vi "PCB name at location.vi"(0 "PCB Outlines in":T1(array[cluster]), 1 "XY Graph":refnum<vi>, 7 "XY":cluster{"X":dbl, "Y":dbl}, 11 "error in":errorcluster) -> (4 "PCB Outlines out":T1(array[cluster]), 6 "PCB Name":string, 8 "Outline mean":cluster{"X":dbl, "Y":dbl}, 10 "Within outline":bool, 14 "x y position":cluster{"X":dbl, "Y":dbl}, 15 "error out":errorcluster)   [LabVIEW 2013, in "Manipulate IPF.lvlib"]
uses:
  <vilib>/Analysis/baseanly.llb/Mean (DBL).vi
  <vilib>/Analysis/geometry.llb/Point in Polygon (Scalar).vi
  Manipulate IPF.lvlib
  <vilib>/Analysis/NI_AAL_Geometry.lvlib
  <vilib>/Analysis/NI_AALBase.lvlib
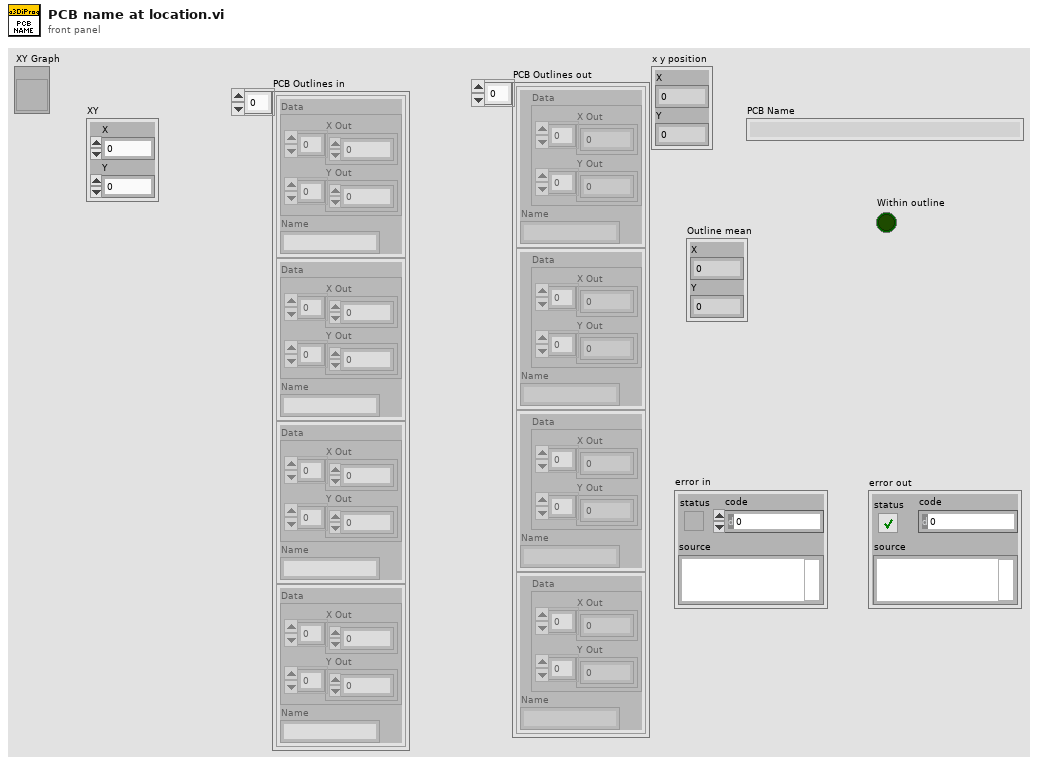
[diagram p1: front panel]
types:
  T1 = cluster{"Data":cluster{"X Out":dbl[], "Y Out":dbl[]}, "Name":string}[]
  T2 = cluster{"Data":cluster{"X Out":dbl[], "Y Out":dbl[]}, "Name":string}
  T3 = typedef "NI_AAL_Geometry.lvlib/Point in Polygon Position.ctl" = u16
  T4 = typedef "LVPoint32TypeDef.ctl" = cluster{"Horizontal":i32, "Vertical":i32}
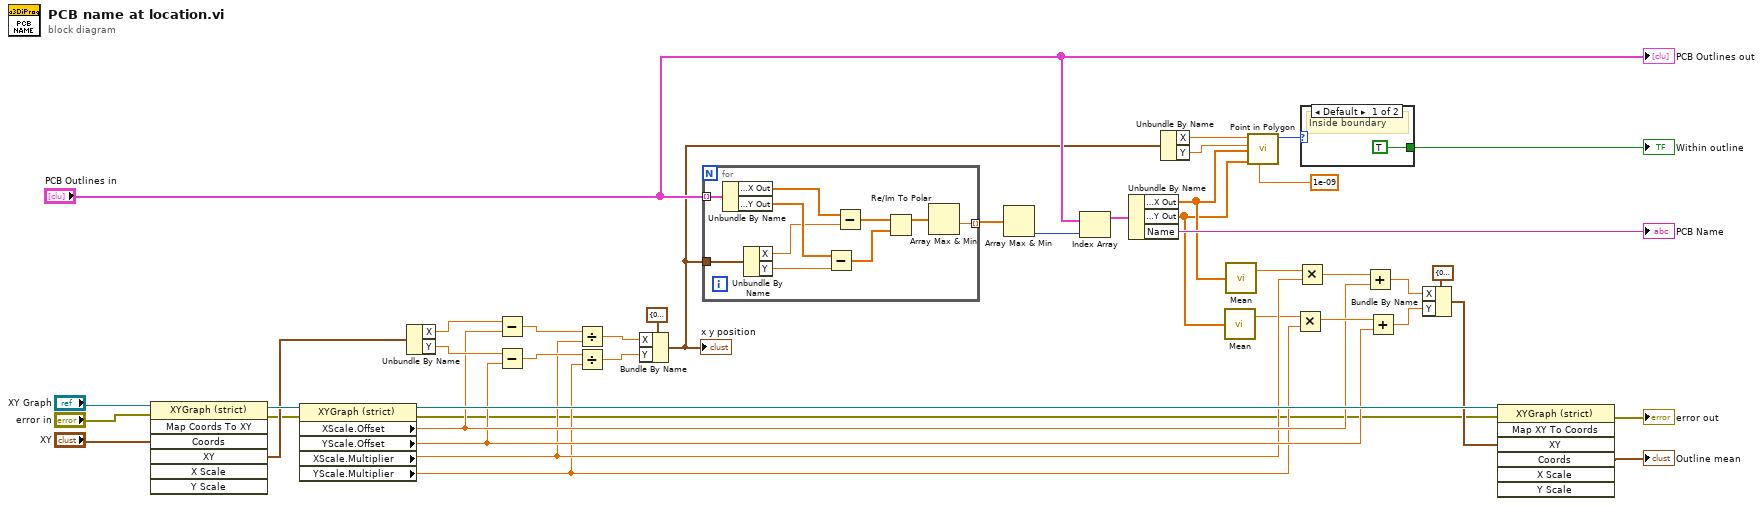
[diagram p0: block diagram]
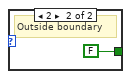
[diagram p2: hidden frame]
diagram:
  n1 = invoke class="XYGraph (strict)" method="Map Coords To XY"(reference="XY Graph", error in="error in", "Coords"="XY") -> (reference out=w22:refnum<vi>, error out=w7:errorcluster, "XY"=w19:cluster{"X":dbl, "Y":dbl})  [unwired: 4 in, 4 out]
  n2 = property on="Property Node" class="XYGraph (strict)"(reference=w22, error in=w7) -> (reference out=w21:refnum<vi>, error out=w9:errorcluster, "XScale.Offset"=w14:dbl, "YScale.Offset"=w13:dbl, "XScale.Multiplier"=w12:dbl, "YScale.Multiplier"=w11:dbl)
  n3 = Unbundle By Name(w19) -> ("X"=w26:dbl, "Y"=w30:dbl)
  n4 = Subtract(x=w26, y=w14) -> (x-y=w29:dbl)
  n5 = Subtract(x=w30, y=w13) -> (x-y=w31:dbl)
  n6 = Divide(x=w29, y=w12) -> (x/y=w28:dbl)
  n7 = Divide(x=w31, y=w11) -> (x/y=w27:dbl)
  n8 = Bundle By Name(cluster=cluster{"X":dbl, "Y":dbl} {"X"=0.0, "Y"=0.0} ("XY"), "X"=w28, "Y"=w27) -> (w24:cluster{"X":dbl, "Y":dbl})
  "x y position" <- w24
  n9 = for {
    tunnel: w24 -> [w51]
    tunnel: "PCB Outlines in" -> [w52] mode=indexing
    tunnel: [w49] -> w42 mode=indexing
    n10 = Unbundle By Name(w52) -> ("Data.X Out"=w47:dbl[], "Data.Y Out"=w48:dbl[])
    n11 = Unbundle By Name(w51) -> ("X"=w45:dbl, "Y"=w46:dbl)
    n12 = Subtract(x=w48, y=w46) -> (x-y=w43:dbl[])
    n13 = Subtract(x=w47, y=w45) -> (x-y=w44:dbl[])
    n14 = Re/Im To Polar(2:w43, 3:w44) -> (1:w50:dbl[])  [unwired: 1 out]
    n15 = Array Max & Min(array=w50) -> (min value=w49:dbl)  [unwired: 3 out]
  }
  n16 = Array Max & Min(array=w42) -> (min index (indices)=w41:i32)  [unwired: 3 out]
  n17 = Index Array(array="PCB Outlines in", index=w41) -> (element=w39:T2)
  n18 = Unbundle By Name(w39) -> ("Data.X Out"=w6:dbl[], "Data.Y Out"=w5:dbl[], "Name"=→"PCB Name":string)
  n19 = Unbundle By Name(w24) -> ("X"=w37:dbl, "Y"=w36:dbl)
  n20 = call-poly <vilib>:"Mean.vi"("X"=w5) -> ("mean"=w1:dbl)  [unwired: 1 out]
  n21 = call-poly <vilib>:"Mean.vi"("X"=w6) -> ("mean"=w2:dbl)  [unwired: 1 out]
  n22 = call-poly <vilib>:"Point in Polygon.vi"("tolerance"=1e-09, "Polygon Y"=w5, "Polygon X"=w6, "y"=w36, "x"=w37) -> ("position"=w34:T3)  [unwired: 5 in, 1 out]
  n23 = Multiply(x=w1, y=w11) -> (x*y=w15:dbl)
  n24 = Multiply(x=w2, y=w12) -> (x*y=w16:dbl)
  n25 = case shown="Default" w34 {
    tunnel: [TRUE FALSE] -> w33
    frame Default {
      # "Inside boundary"
    }
    frame 2 {
      # "Outside boundary"
    }
  }
  "Within outline" <- w33
  n26 = Add(x=w16, y=w14) -> (x+y=w4:dbl)
  n27 = Add(x=w15, y=w13) -> (x+y=w3:dbl)
  n28 = Bundle By Name(cluster=cluster{"X":dbl, "Y":dbl} {"X"=0.0, "Y"=0.0} ("XY"), "X"=w4, "Y"=w3) -> (w17:cluster{"X":dbl, "Y":dbl})
  n29 = invoke class="XYGraph (strict)" method="Map XY To Coords"(reference=w21, error in=w9, "XY"=w17) -> (error out=→"error out":errorcluster, "Coords"=→"Outline mean":T4)  [unwired: 4 in, 5 out]
  "PCB Outlines out" <- "PCB Outlines in"
